vi "NavDisplay Handler.vi"(7 "Roll":i32, 8 "roll image":T1, 9 "Pitch":i32, 10 "pitch image":T1) -> (3 "new picture":picture)   [LabVIEW 2009]
uses:
  <vilib>/picture/picture.llb/imagedata.ctl
  GCS26/Rotate.llb/rotate 24bit.vi
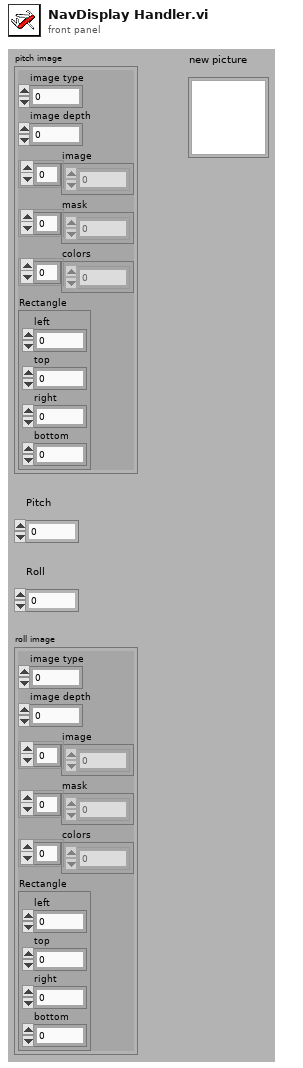
[diagram p1: front panel]
types:
  T1 = typedef "imagedata.ctl" = cluster{"image type":i32, "image depth":i32, "image":u8[], "mask":u8[], "colors":u32[], "Rectangle":cluster{"left":i16, "top":i16, "right":i16, "bottom":i16}}
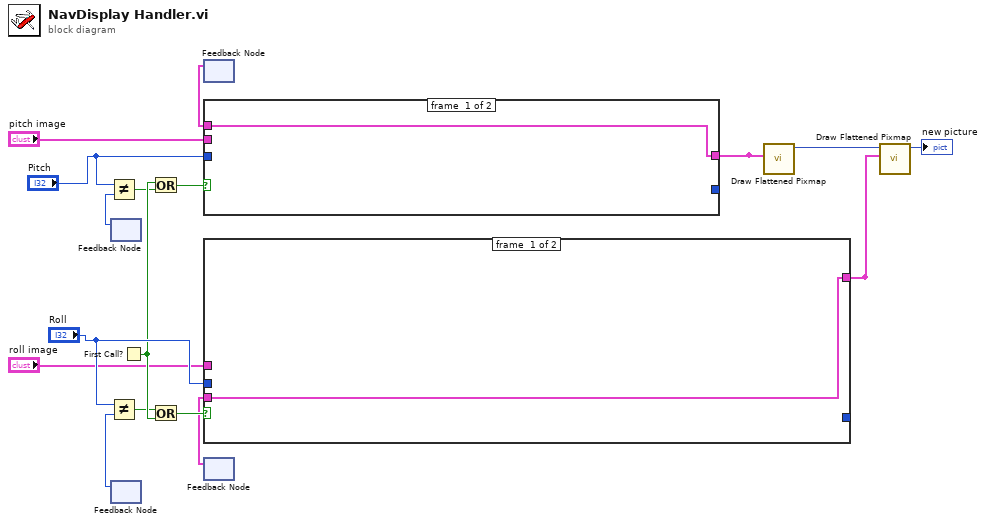
[diagram p0: block diagram]
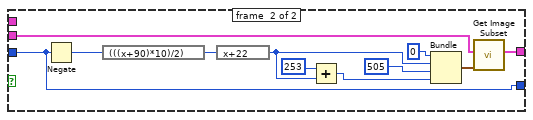
[diagram p2: hidden frame]
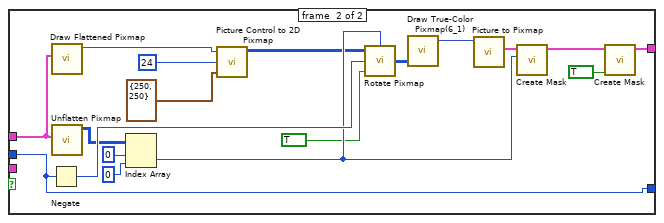
[diagram p3: hidden frame]
diagram:
  n1 = feedback #1() -> (w7:i32)  [unwired: 1 out]
  n2 = Not Equal?(x="Pitch", y=w7) -> (x != y?=w13:bool)
  n3 = feedback #2() -> (w2:i32)  [unwired: 1 out]
  n4 = Not Equal?(x="Roll", y=w2) -> (x != y?=w12:bool)
  n5 = First Call?() -> (First Call?: T/F=w16:bool)
  n6 = Or(x=w16, y=w13) -> (x .or. y?=w15:bool)
  n7 = Or(x=w12, y=w16) -> (x .or. y?=w14:bool)
  n8 = feedback #3() -> (w9:T1)  [unwired: 1 out]
  n9 = case shown="True" w15 {
    tunnel: "pitch image" -> [_ w31]
    tunnel: "Pitch" -> [_ w21]
    tunnel: [w20 w22] -> w8
    tunnel: [_ w21] -> w6
    tunnel: w9 -> [w20 _]
    frame #0 {
    }
    frame #1 {
      n10 = Negate(x=w21) -> (-x=w23:i32)
      n11 = expression code="(((x+90)*10)/2)"(w23) -> (w24:i32)
      n12 = expression code="x+22"(w24) -> (w25:i32)
      n13 = Add(x=253, y=w25) -> (x+y=w26:i32)
      n14 = Bundle(0, w25, 505, w26) -> (w30:cluster{i32, i32, i32, i32})  [unwired: 1 out]
      n15 = call <vilib>:"Get Image Subset.vi"("subset rect"=w30, "image data"=w31) -> ("image subset"=w22:T1)  [unwired: 5 out]
    }
  }
  n16 = feedback #4() -> (w4:T1)  [unwired: 1 out]
  n17 = case shown="True" w14 {
    tunnel: "Roll" -> [_ w36]
    tunnel: "roll image" -> [_ w35]
    tunnel: [_ w36] -> w1
    tunnel: [w32 w33] -> w3
    tunnel: w4 -> [w32 _]
    frame #0 {
    }
    frame #1 {
      n18 = Negate(x=w36) -> (-x=w50:i32)
      n19 = call <vilib>:"Draw Flattened Pixmap.vi"("image data"=w35) -> ("new picture"=w34:picture)  [unwired: 1 in, 7 out]
      n20 = call <vilib>:"Unflatten Pixmap.vi"("image data"=w35) -> ("24-bit pixmap"=w39:u32[][])  [unwired: 10 out]
      n21 = Index Array(array=w39, index (row)=0, index (col)=0 ("disabled index (col)")) -> (element=w47:u32)
      n22 = call "Picture Control to 2D Pixmap.vi"("Picture"=w34, "image depth"=u8 24, "Draw Area Size"=cluster{"Width":u32, "Height":u32} {"Width"=250, "Height"=250}) -> ("24-bit"=w41:u32[][])  [unwired: 4 out]
      n23 = call-poly "Rotate Pixmap.vi"("Color Table Index of Fill Color"=w47, "Maintain Center Position?"=TRUE, "Rotation Angle (degrees)"=w50, "Pixmap"=w41) -> ("Rotated Pixmap"=w45:u32[][])
      n24 = call <vilib>:"Draw True-Color Pixmap(6_1).vi"("data (RGB format)"=w45) -> ("new picture"=w38:picture)  [unwired: 2 in, 6 out]
      n25 = call <vilib>:"Picture to Pixmap.vi"("picture"=w38) -> ("image data"=w46:T1)  [unwired: 3 in, 7 out]
      n26 = call <vilib>:"Create Mask.vi"("Mask Color (Black)"=w47, "image data"=w46) -> ("image data"=w48:T1)  [unwired: 2 in, 7 out]
      n27 = call <vilib>:"Create Mask.vi"("Combine Masks? (F)"=TRUE, "image data"=w48) -> ("image data"=w33:T1)  [unwired: 2 in, 7 out]
    }
  }
  n28 = call <vilib>:"Draw Flattened Pixmap.vi"("image data"=w8) -> ("new picture"=w5:picture)  [unwired: 1 in, 7 out]
  n29 = call <vilib>:"Draw Flattened Pixmap.vi"("image data"=w3, "picture"=w5) -> ("new picture"=→"new picture":picture)  [unwired: 7 out]
